vi "ImPro - Apply to All Images.vi"(7 "ImProSettings Current":T1, 8 "error in (no error)":errorcluster, 9 "Rectangle":T3, 10 "24-bit pixmap":u32[][](array[numeric]), 11 "UI Refs":T2) -> (0 "error out":errorcluster, 5 "ImProSettings NEW":T1)   [LabVIEW 2023]
uses:
  Controls/ImPro - UI Refs.ctl
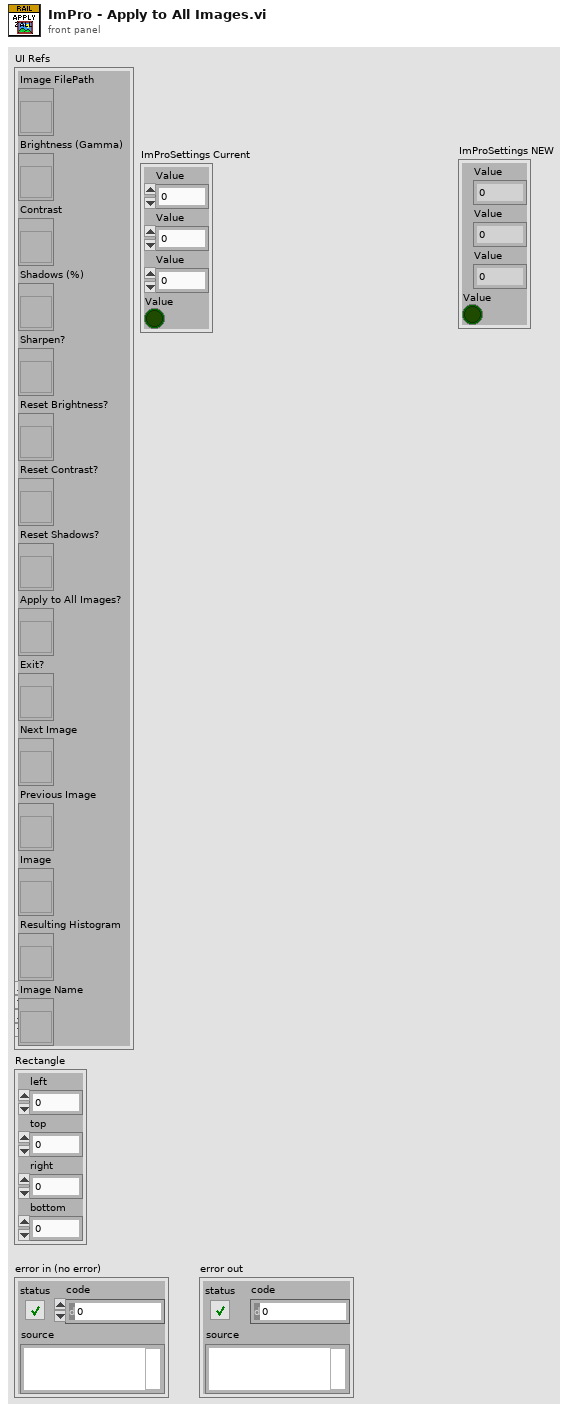
[diagram p1: front panel]
types:
  T1 = cluster{"Value":dbl, "Value":dbl, "Value":dbl, "Value":bool}
  T2 = typedef "ImPro - UI Refs.ctl" = cluster{"Image FilePath":refnum<vi>, "Brightness (Gamma)":refnum<vi>, "Contrast":refnum<vi>, "Shadows (%)":refnum<vi>, "Sharpen?":refnum<vi>, "Reset Brightness?":refnum<vi>, "Reset Contrast?":refnum<vi>, "Reset Shadows?":refnum<vi>, "Apply to All Images?":refnum<vi>, "Exit?":refnum<vi>, "Next Image":refnum<vi>, "Previous Image":refnum<vi>, "Image":refnum<vi>, "Resulting Histogram":refnum<vi>, "Image Name":refnum<vi>}
  T3 = cluster{"left":i16, "top":i16, "right":i16, "bottom":i16}
  T4 = cluster{"Brightness":dbl, "Contrast":dbl, "Shadows":dbl, "Sharpen?":bool}
  T5 = typedef "imagedata.ctl" = cluster{"image type":i32, "image depth":i32, "image":u8[], "mask":u8[], "colors":u32[], "Rectangle":cluster{"left":i16, "top":i16, "right":i16, "bottom":i16}}
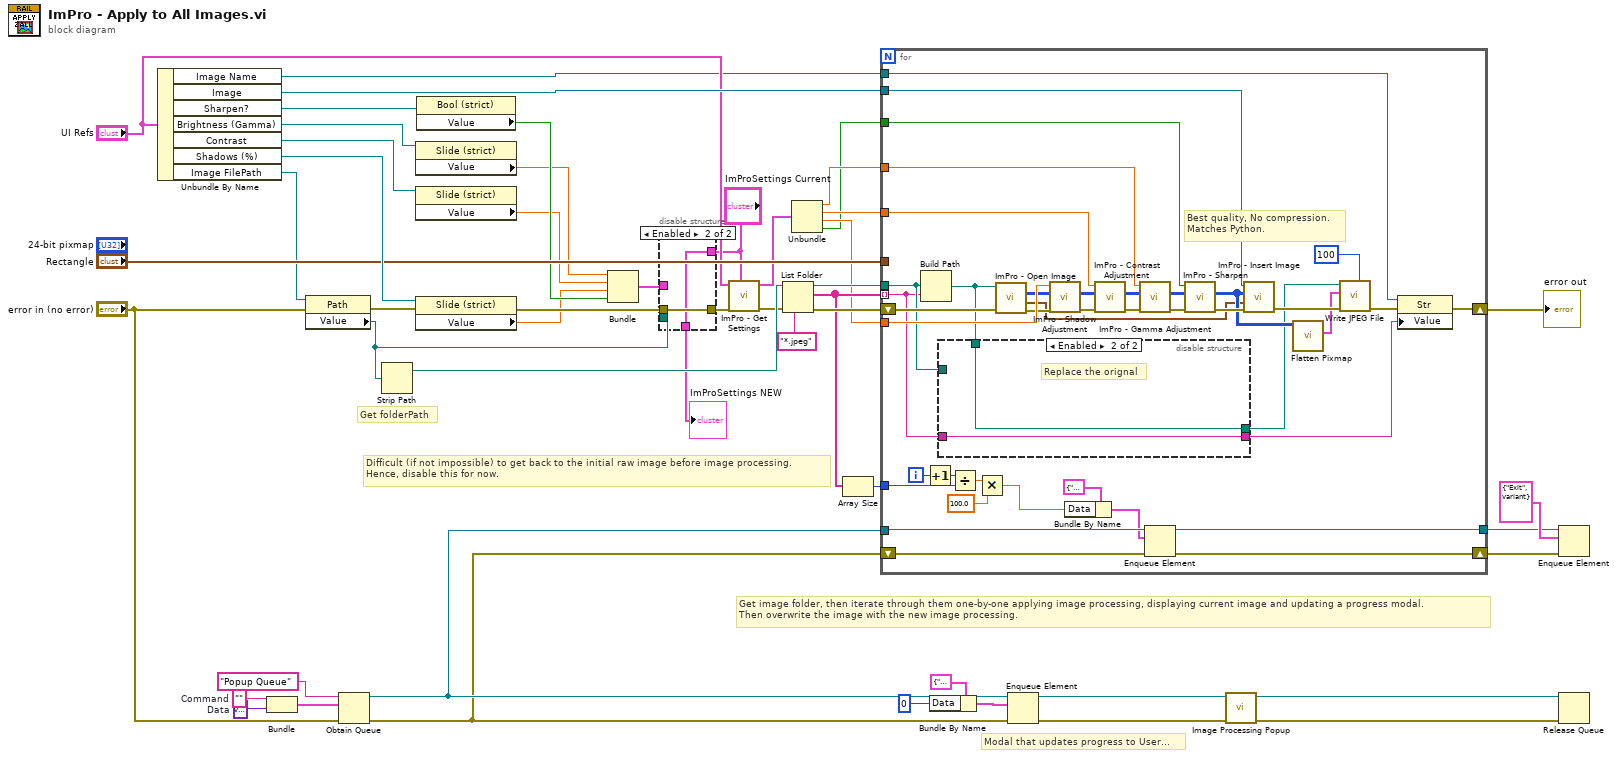
[diagram p0: block diagram]
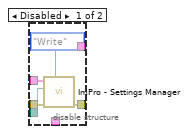
[diagram p2: hidden frame]
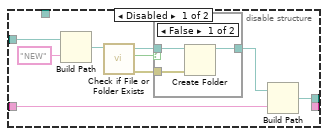
[diagram p3: hidden frame]
diagram:
  w33 = variant  # Data
  w36 = ""  # Command
  # "Difficult (if not impossible) to get back to the initial raw image before image processing.\nHence, disable this for now."
  # "Modal that updates progress to User..."
  # "Get folderPath"
  # "Get image folder, then iterate through them one-by-one applying image processing, displaying current image and updating a progress modal.\nThen overwrite the image with the new image processing."
  n1 = Unbundle By Name("UI Refs") -> ("Image Name"=w1:refnum<vi>, "Image"=w49:refnum<vi>, "Sharpen?"=w50:refnum<vi>, "Brightness (Gamma)"=w48:refnum<vi>, "Contrast"=w47:refnum<vi>, "Shadows (%)"=w46:refnum<vi>, "Image FilePath"=w43:refnum<vi>)
  n2 = Bundle("Command"=w36, "Data"=w33) -> (w32:cluster{"Command":string, "Data":variant})  [unwired: 1 in]
  n3 = property class="Path"(reference=w43, error in="error in (no error)") -> (error out=w44:errorcluster, "Value"=w18:path)  [unwired: 1 out]
  n4 = Obtain Queue(name (unnamed)="Popup Queue", element data type=w32, error in (no error)="error in (no error)") -> (queue out=w29:refnum<queue>, error out=w24:errorcluster)  [unwired: 2 in, 1 out]
  n5 = Strip Path(path=w18) -> (stripped path=w41:path)  [unwired: 1 out]
  n6 = property class="Slide (strict)"(reference=w48) -> ("Value"=w14:dbl)  [unwired: 1 in, 2 out]
  n7 = property class="Slide (strict)"(reference=w47) -> ("Value"=w15:dbl)  [unwired: 1 in, 2 out]
  n8 = property class="Slide (strict)"(reference=w46, error in=w44) -> (error out=w19:errorcluster, "Value"=w16:dbl)  [unwired: 1 out]
  n9 = property class="Bool (strict)"(reference=w50) -> ("Value"=w17:bool)  [unwired: 1 in, 2 out]
  n10 = Bundle("Value"=w14, "Value"=w15, "Value"=w16, "Value"=w17) -> (w6:T1)  [unwired: 1 in]
  n11 = disable-structure shown="Enabled" {
    disable-tunnel: w19 -> [w54 w57]
    disable-tunnel: w6 -> [w53 _]
    disable-tunnel: w18 -> [w52 _]
    disable-tunnel: [w51 w57] -> w12
    disable-tunnel: [_ w56] -> w3
    disable-tunnel: "ImProSettings Current" -> [_ w56]
    frame Disabled {
      n12 = call "ImPro - Settings Manager.vi"("Command"=enum16{"Read", "Write"}."Write", "error in (no error)"=w54, "ImagePath"=w52, "ImProSettings In"=w53) -> ("error out"=w51:errorcluster)  [unwired: 6 in, 1 out]
    }
    frame Enabled {
    }
  }
  "ImProSettings NEW" <- w3
  n13 = call "ImPro - Get Settings.vi"("ImProSettings on File"="ImProSettings Current", "error in (no error)"=w12, "output cluster"="UI Refs") -> ("error out"=w11:errorcluster, "ImProSettings Relative"=w4:T4)  [unwired: 7 in]
  n14 = List Folder(path=w41, pattern="*.jpeg", error in=w11) -> (path out=w40:path, filenames=w39:string[], error out=w42:errorcluster)  [unwired: 1 in, 1 out]
  n15 = Unbundle(w4) -> ("Brightness"=w8:dbl, "Contrast"=w9:dbl, "Shadows"=w10:dbl, "Sharpen?"=w7:bool)
  n16 = Array Size(array=w39) -> (size(s)=w38:i32)
  n17 = for {
    tunnel: w7 -> [w97]
    tunnel: w49 -> [w96]
    tunnel: w8 -> [w92]
    tunnel: w9 -> [w91]
    tunnel: w10 -> [w90]
    tunnel: "Rectangle" -> [_]
    shift-right: [w60] -> w20
    shift-left: w42 -> [w85]
    tunnel: w39 -> [w75] mode=indexing
    tunnel: w40 -> [w76]
    tunnel: w38 -> [w72]
    tunnel: w29 -> [w68]
    tunnel: [w64] -> w26
    shift-right: [w63] -> w25
    shift-left: w24 -> [w62]
    tunnel: w1 -> [w59]
    i -> [w73]
    # "Best quality, No compression.\nMatches Python."
    n18 = Build Path(base path=w76, name or relative path=w75) -> (appended path=w61:path)
    n19 = Increment(x=w73) -> (x+1=w71:i32)
    n20 = disable-structure shown="Enabled" {
      disable-tunnel: w76 -> [w106 _]
      disable-tunnel: w75 -> [w104 w111]
      disable-tunnel: [w103 w112] -> w74
      disable-tunnel: w61 -> [_ w112]
      disable-tunnel: [_ w111] -> w58
      frame Disabled {
        n21 = Build Path(base path=w106, name or relative path="NEW") -> (appended path=w102:path)
        n22 = call <vilib>:"Check if File or Folder Exists.vi"("path"=w102) -> ("error out"=w100:errorcluster, "file or folder exists?"=w99:bool, "dup path"=w101:path)  [unwired: 8 in]
        n23 = case shown="False" w99 {
          tunnel: w101 -> [w109 w110]
          tunnel: w100 -> [w108 _]
          tunnel: [w107 w110] -> w98
          frame False {
            n24 = Create Folder(path (use dialog)=w109, error in=w108) -> (created path=w107:path)  [unwired: 1 in, 2 out]
          }
          frame True {
          }
        }
        n25 = Build Path(base path=w98, name or relative path=w104) -> (appended path=w103:path)
      }
      frame Enabled {
        # "Replace the orignal"
      }
    }
    n26 = Divide(x=w71, y=w72) -> (x/y=w70:dbl)
    n27 = Multiply(x=w70, y=100.0) -> (x*y=w66:dbl)
    n28 = call "ImPro - Open Image.vi"("error in (no error)"=w85, "path to PNG file"=w61) -> ("error out"=w84:errorcluster, "Rectangle"=w78:T3, "24-bit pixmap"=w83:u32[][])  [unwired: 6 in, 1 out]
    n29 = call "ImPro - Shadow Adjustment.vi"("error in (no error)"=w84, "24-bit pixmap In"=w83, "Shadows (%)"=w90) -> ("error out"=w87:errorcluster, "24-bit pixmap Out"=w86:u32[][])  [unwired: 6 in, 1 out]
    n30 = Bundle By Name(cluster=cluster{"Command":string, "Data":variant} {"Command"="Update Progress", "Data"=variant} ("output cluster"), "Data"=w66) -> (w65:cluster{"Command":string, "Data":variant})
    n31 = call "ImPro - Contrast Adjustment.vi"("error in (no error)"=w87, "24-bit pixmap In"=w86, "Contrast"=w91) -> ("error out"=w88:errorcluster, "24-bit pixmap Out"=w89:u32[][])  [unwired: 7 in]
    n32 = call "ImPro - Gamma Adjustment.vi"("error in (no error)"=w88, "24-bit pixmap In"=w89, "Brightness (Gamma)"=w92) -> ("error out"=w93:errorcluster, "24-bit pixmap Out"=w94:u32[][])  [unwired: 6 in, 1 out]
    n33 = Enqueue Element(queue=w68, element=w65, error in (no error)=w62) -> (queue out=w64:refnum<queue>, error out=w63:errorcluster)  [unwired: 1 in, 1 out]
    n34 = call "ImPro - Sharpen.vi"("error in (no error)"=w93, "24-bit pixmap In"=w94, "Sharpen?"=w97) -> ("error out"=w95:errorcluster, "24-bit pixmap Out"=w79:u32[][])  [unwired: 7 in]
    n35 = call "ImPro - Insert Image.vi"("error in (no error)"=w95, "Rectangle"=w78, "24-bit pixmap"=w79, "Picture in"=w96) -> ("error out"=w82:errorcluster)  [unwired: 7 in]
    n36 = call <vilib>:"Flatten Pixmap.vi"("24-bit pixmap"=w79) -> ("image data"=w77:T5)  [unwired: 10 in]
    n37 = call <vilib>:"Write JPEG File.vi"("quality (80)"=100, "error in (no error)"=w82, "image data"=w77, "path to JPEG file"=w74) -> ("error out"=w81:errorcluster)  [unwired: 6 in, 1 out]
    n38 = property class="Str"(reference=w59, error in=w81, "Value"=w58) -> (error out=w60:errorcluster)  [unwired: 1 out]
  }
  "error out" <- w20
  n39 = Bundle By Name(cluster=cluster{"Command":string, "Data":variant} {"Command"="Update Progress", "Data"=variant} ("output cluster"), "Data"=u8 0 ("Progress")) -> (w35:cluster{"Command":string, "Data":variant})
  n40 = Enqueue Element(queue=w29, element=w35, error in (no error)=w24) -> (queue out=w22:refnum<queue>, error out=w28:errorcluster)  [unwired: 1 in, 1 out]
  n41 = call "Image Processing Popup.vi"("error in"=w28, "queue in"=w22) -> ("error out"=w23:errorcluster, "queue out"=w21:refnum<queue>)  [unwired: 8 in]
  n42 = Enqueue Element(queue=w26, element=cluster{"Command":string, "Data":variant} {"Command"="Exit", "Data"=variant} ("output cluster"), error in (no error)=w25) -> ()  [unwired: 1 in, 3 out]
  n43 = Release Queue(queue=w21, error in (no error)=w23) -> ()  [unwired: 1 in, 3 out]
